vi "CloseAlllHandles.vi"(8 "error in (no error)":errorcluster, 11 "Handles_In":T1) -> (0 "error out":errorcluster, 3 "Handles_Out":T1)   [LabVIEW 2017]
uses:
  InstrumentsInterfaces/Motordriver/maxon EPOS/Examples/maxonEPOS.lvlib
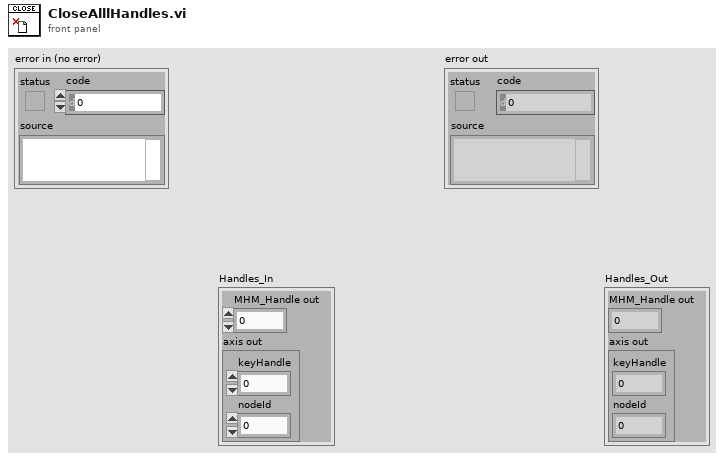
[diagram p1: front panel]
types:
  T1 = cluster{"MHM_Handle out":u32, "axis out":cluster{"keyHandle":u32, "nodeId":u16}}
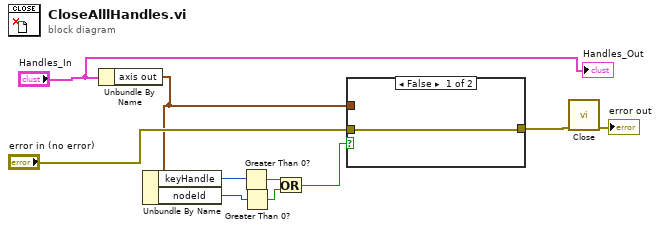
[diagram p0: block diagram]
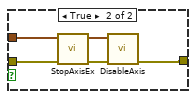
[diagram p2: hidden frame]
diagram:
  n1 = Unbundle By Name("Handles_In") -> ("axis out"=w6:cluster{"keyHandle":u32, "nodeId":u16})
  n2 = Unbundle By Name(w6) -> ("keyHandle"=w5:u32, "nodeId"=w4:u16)
  n3 = Greater Than 0?(x=w5) -> (x > 0?=w3:bool)
  n4 = Greater Than 0?(x=w4) -> (x > 0?=w2:bool)
  n5 = Or(x=w3, y=w2) -> (x .or. y?=w1:bool)
  n6 = case shown="False" w1 {
    tunnel: [w11 w15] -> w10
    tunnel: "error in (no error)" -> [w11 w13]
    tunnel: w6 -> [_ w12]
    frame False {
    }
    frame True {
      n7 = call "StopAxisEx.vi"("error in (no error)"=w13, "axis in"=w12) -> ("error out"=w14:errorcluster, "axis out"=w16:cluster{"keyHandle":u32, "nodeId":u16})  [unwired: 4 in]
      n8 = call "DisableAxis.vi"("error in (no error)"=w14, "axis in"=w16) -> ("error out"=w15:errorcluster)  [unwired: 4 in, 1 out]
    }
  }
  n9 = call "Close.vi"("error in (no error)"=w10) -> ("error out"=→"error out":errorcluster)  [unwired: 10 in]
  "Handles_Out" <- "Handles_In"
